vi "SysLog Status.vi"() -> ()   [LabVIEW 2020, in "SysLog.lvlib"]
uses:
  SysLog.lvlib
  Visualisierungs Elemente/Button.ctl
  Aktionen FGV SysLog.ctl
  Allgemein/allgemeine Sub-VIs.lvlib
panel:
  in  "Schieberegler":i32(slide) caption="Transparenz" min=0 max=70 step=1 scale=0.0..100.0
  in  "SysLogHistory":T1
  in  "SystemLogListe":i32[](listbox)
  # "System Log Status"
  # "System Log Meldungen werden hier nur vorübergehend als Status angezeigt und dann in die History Datei geschrieben, und dient daher nur zum aktuellen Überblick.\nBitte die SysLogHistorie öffnen für eine umfangreiche Recherche."
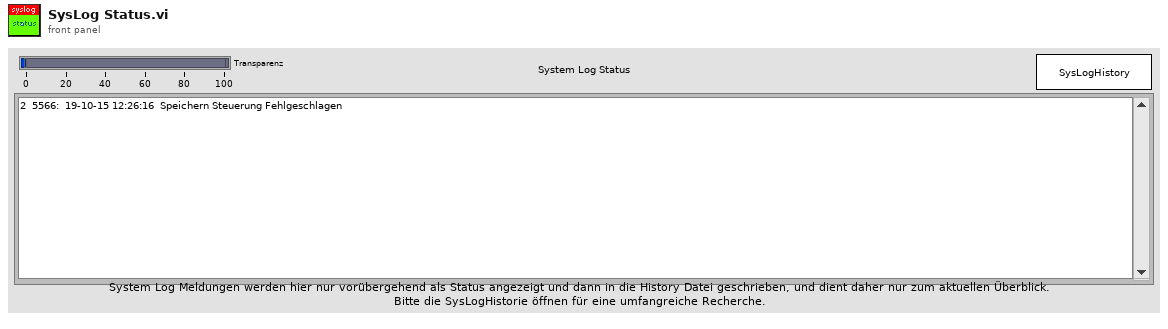
[diagram p1: front panel]
types:
  T1 = typedef "Button.ctl" = bool
  T2 = typedef "SysLog.lvlib/Aktionen FGV SysLog.ctl" = enum16{"initialisieren", "lesen", "schreiben", "history button ref", "Syslog_Anforderung"}
  T3 = cluster{"Anzeige Array":bool[], "Message Array":string[], "SysLog Incon Array":enum16{"OK", "Warnung", "Fehler"}[], "Status Message Array":string[], "Status SysLog Incon Array":enum16{"OK", "Warnung", "Fehler"}[]}
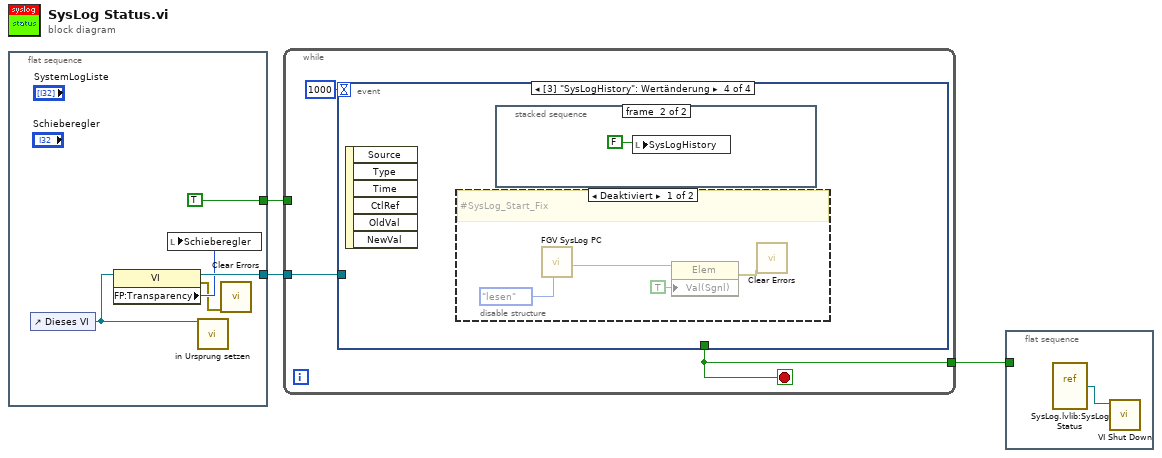
[diagram p0: block diagram]
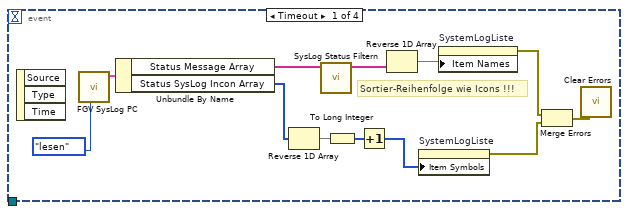
[diagram p2: hidden frame]
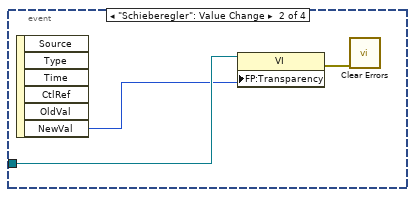
[diagram p3: hidden frame]
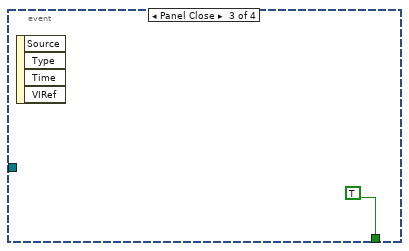
[diagram p4: hidden frame]
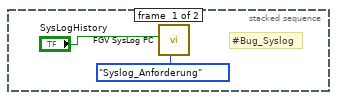
[diagram p5: hidden frame]
diagram:
  n1 = flat-sequence {
    tunnel: [TRUE] -> w2
    tunnel: [w6] -> w1
    frame #0 {
      n2 = control-ref of="Dieses VI"() -> (w6:refnum<vi>)
      n3 = property class="VI"(reference=w6) -> (error out=w4:errorcluster, "FP:Transparency"=w5:u8)  [unwired: 1 in, 1 out]
      n4 = local write "Schieberegler"(w5) -> ()
      n5 = call "in Ursprung setzen.vi"("VI Referenz"=w6) -> ()  [unwired: 10 in, 1 out]
      n6 = call <vilib>:"Clear Errors.vi"("error in (no error)"=w4) -> ()  [unwired: 5 in, 2 out]
    }
  }
  n7 = while {
    tunnel: [w9] -> w3
    tunnel: w2 -> [_]
    tunnel: w1 -> [w8]
    stop <- w9 stop-if-true
    n8 = event shown="[3] \"SysLogHistory\": Wertänderung" {
      selector: _ -> [_ _ _ _]
      dyn-events: _ -> [_ _ _ _]
      timeout: 1000 -> [_ _ _ _]
      tunnel: [_ _ TRUE _] -> w9
      tunnel: w8 -> [_ w25 _ _]
      event Timeout {
        # "Sortier-Reihenfolge wie Icons !!!"
        n9 = event-data() -> ()  [unwired: 1 in, 3 out]
        n10 = call "FGV SysLog PC.vi"("Aktion"=Aktionen_FGV_SysLog."lesen") -> ("Anzeige Cluster"=w13:T3)  [unwired: 6 in, 4 out]
        n11 = Unbundle By Name(w13) -> ("Status Message Array"=w12:string[], "Status SysLog Incon Array"=w11:enum16{"OK", "Warnung", "Fehler"}[])
        n12 = Reverse 1D Array(array=w11) -> (reversed array=w20:enum16{"OK", "Warnung", "Fehler"}[])
        n13 = call "SysLog Status Filtern.vi"("Message Array"=w12) -> ("Message Array"=w18:string[])  [unwired: 10 in]
        n14 = To Long Integer(number=w20) -> (32bit integer=w21:i32[])
        n15 = Increment(x=w21) -> (x+1=w19:i32[])
        n16 = Reverse 1D Array(array=w18) -> (reversed array=w17:string[])
        n17 = property on="SystemLogListe" class="Listenfeld (strikt)"("Item Symbols"=w19) -> (error out=w14:errorcluster)  [unwired: 2 in, 1 out]
        n18 = property on="SystemLogListe" class="Listenfeld (strikt)"("Item Names"=w17) -> (error out=w15:errorcluster)  [unwired: 2 in, 1 out]
        n19 = Merge Errors(w15, w14) -> (w16:errorcluster)
        n20 = call <vilib>:"Clear Errors.vi"("error in (no error)"=w16) -> ()  [unwired: 5 in, 2 out]
      }
      event "Schieberegler": Value Change {
        n21 = event-data() -> ("NewVal"=w24:i32)  [unwired: 1 in, 5 out]
        n22 = property class="VI"(reference=w25, "FP:Transparency"=w24) -> (error out=w23:errorcluster)  [unwired: 1 in, 1 out]
        n23 = call <vilib>:"Clear Errors.vi"("error in (no error)"=w23) -> ()  [unwired: 5 in, 2 out]
      }
      event Panel Close {
        n24 = event-data() -> ()  [unwired: 1 in, 4 out]
      }
      event Value Change {
        n25 = event-data() -> ()  [unwired: 1 in, 6 out]
        n26 = disable-structure shown="Deaktiviert" {
          frame Disabled {
            # "#SysLog_Start_Fix"
            n27 = call "FGV SysLog PC.vi"("Aktion"=Aktionen_FGV_SysLog."lesen") -> ("Main History Button Referenz out"=w31:refnum<vi>)  [unwired: 6 in, 4 out]
            n28 = property class="Elem"(reference=w31, "Val(Sgnl)"=TRUE) -> (error out=w33:errorcluster)  [unwired: 1 in, 1 out]
            n29 = call <vilib>:"Clear Errors.vi"("error in (no error)"=w33) -> ()  [unwired: 5 in, 2 out]
          }
          frame Enabled {
          }
        }
        n30 = stacked-sequence {
          frame #0 {
            # "#Bug_Syslog"
            n31 = call "FGV SysLog PC.vi"("Aktion"=Aktionen_FGV_SysLog."Syslog_Anforderung", "Syslog Anforderung"="SysLogHistory") -> ()  [unwired: 5 in, 5 out]
          }
          frame #1 {
            n32 = local write "SysLogHistory"(FALSE) -> ()
          }
        }
      }
    }
  }
  n33 = flat-sequence {
    tunnel: w3 -> [_]
    frame #0 {
      n34 = vi-ref "SysLog.lvlib:SysLog Status.vi"() -> (w34:refnum<vi>)
      n35 = call "VI Shut Down.vi"("VI Referenz"=w34) -> ()  [unwired: 11 in]
    }
  }
